vi "Fetch Measurement-Efficiency and Load Reg.vi"(8 "error in":errorcluster, 10 "Measure Call Context in":refnum<class "Measure Call Context.lvclass">, 11 "Efficency fetch measurement":T1={"Load,Source ON&OFF"=0, "Source Ganged Session Out"={"Ganged Config"=enum."Series", "Session List"=[], "Session Mode"=[], "Channel"=[]}, "Load Ganged Session Out"={"Ganged Config"=enum."Series", "Session List"=[], "Session Mode"=[], "Channel"=[]}, "Source sweep values"=[], "Source sweep points"=0, "Load sweep values"=[], "Load sweep points"=0, "Load ganged/single"=FALSE, "Source ganged/single"=FALSE, "Source channel name"="", "Load channel name"="", "Source session out"="", "Load session out"="", "measurement results"={"Source sweep points"=0, "Load sweep points"=0, "Voltage values"=[], "Efficiency"=[], "Ganged load currents"=[], "Ganged load voltages"=[], "Load voltage deviation"=[], "Status"="", "Eload status"=""}, "Nominal output voltage"=0.0, "Measurement timeout"=10.0}) -> (0 "error out":errorcluster, 3 "Efficency fetch measurement":T1={"Load,Source ON&OFF"=0, "Source Ganged Session Out"={"Ganged Config"=enum."Series", "Session List"=[], "Session Mode"=[], "Channel"=[]}, "Load Ganged Session Out"={"Ganged Config"=enum."Series", "Session List"=[], "Session Mode"=[], "Channel"=[]}, "Source sweep values"=[], "Source sweep points"=0, "Load sweep values"=[], "Load sweep points"=0, "Load ganged/single"=FALSE, "Source ganged/single"=FALSE, "Source channel name"="", "Load channel name"="", "Source session out"="", "Load session out"="", "measurement results"={"Source sweep points"=0, "Load sweep points"=0, "Voltage values"=[], "Efficiency"=[], "Ganged load currents"=[], "Ganged load voltages"=[], "Load voltage deviation"=[], "Status"="", "Eload status"=""}, "Nominal output voltage"=0.0, "Measurement timeout"=10.0})   [LabVIEW 2021, in "Eff And Load Reg_Channel Ganging.lvlib"]
doc: "This vi will fetch the measurement in different configuration for and calculate efficiency and load regulation."
uses:
  Eff And Load Reg_Channel Ganging.lvlib
  <vilib>/Plug-In SDKs/Measurements/Measure Call Context/Measure Call Context.lvclass
  Controls/Efficency fetch measurement control.ctl
  shared subVIs/ctl/NIDCPower_channel_ganging - ctl - ganged session.ctl
  shared subVIs/ctl/NIDCPower_channel_ganging - ctl - ganged config.ctl
  shared subVIs/ctl/NIDCPower_channel_ganging - ctl - channel mode.ctl
  Measurement Results.ctl
  <vilib>/Plug-In SDKs/Measurements/Measure Call Context/Accessor/Is Canceled.vi
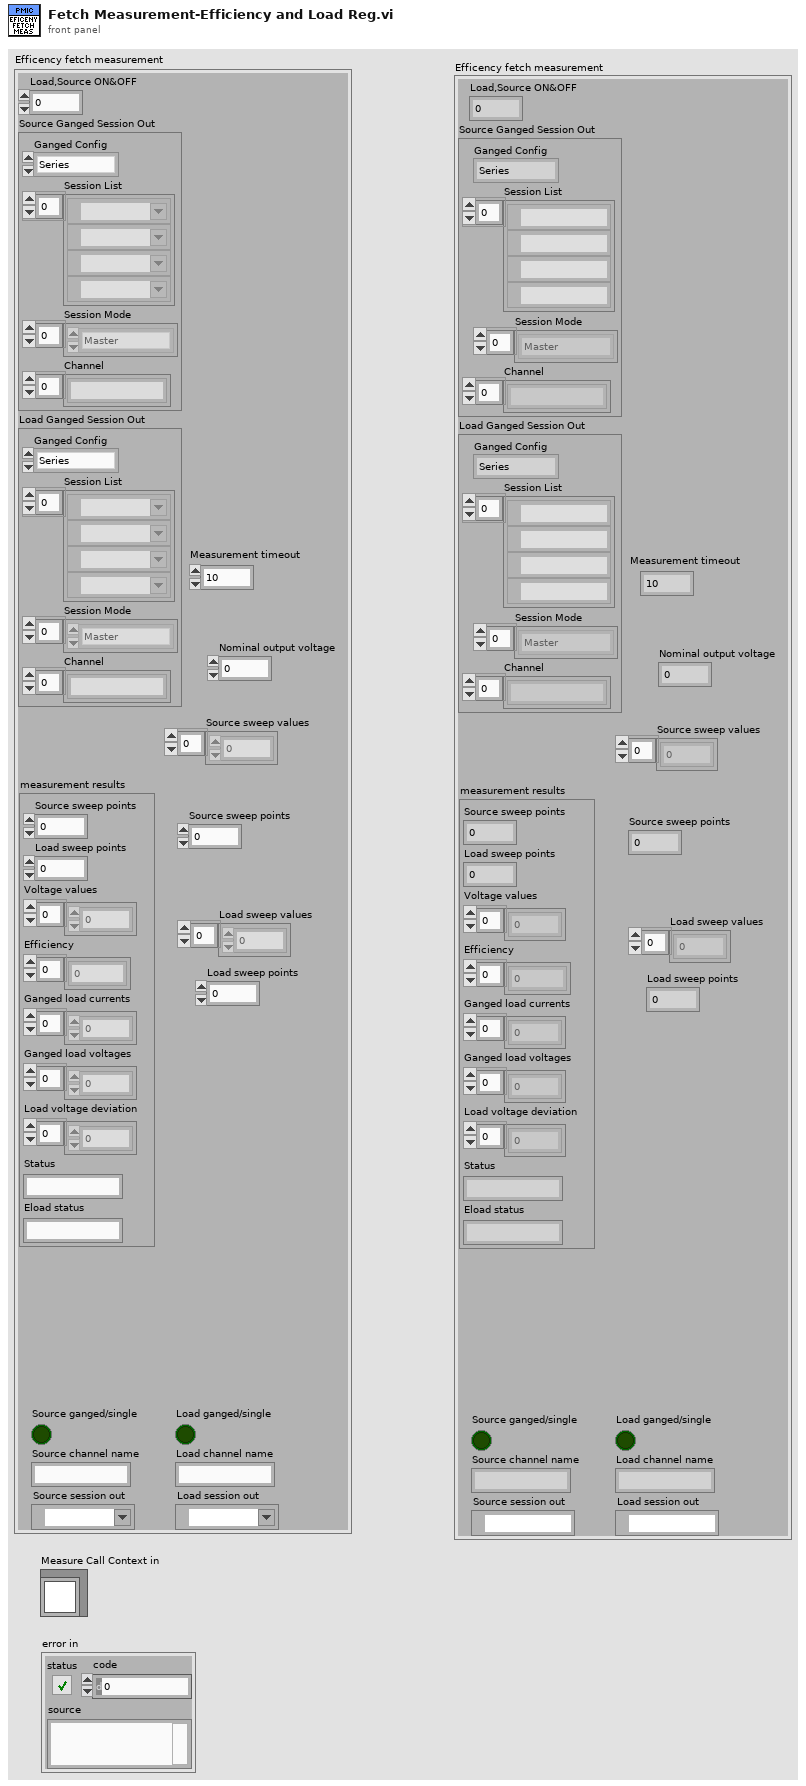
[diagram p1: front panel]
types:
  T1 = typedef "Eff And Load Reg_Channel Ganging.lvlib/Efficency fetch measurement control.ctl" = cluster{"Load,Source ON&OFF":u32, "Source Ganged Session Out":T2, "Load Ganged Session Out":T2, "Source sweep values":dbl[], "Source sweep points":i32, "Load sweep values":dbl[], "Load sweep points":i32, "Load ganged/single":bool, "Source ganged/single":bool, "Source channel name":string, "Load channel name":string, "Source session out":refnum<k15>, "Load session out":refnum<k15>, "measurement results":T5, "Nominal output voltage":dbl, "Measurement timeout":dbl}
  T2 = typedef "NIDCPower_channel_ganging - ctl - ganged session.ctl" = cluster{"Ganged Config":T3, "Session List":refnum<k15>[], "Session Mode":T4[], "Channel":string[]}
  T3 = typedef "NIDCPower_channel_ganging - ctl - ganged config.ctl" = enum32{"Series", "Parallel", "Manual"}
  T4 = typedef "NIDCPower_channel_ganging - ctl - channel mode.ctl" = enum32{"Master", "Slave", "Slave - Inverted"}
  T5 = typedef "Eff And Load Reg_Channel Ganging.lvlib/Measurement Results.ctl" = cluster{"Source sweep points":i32, "Load sweep points":i32, "Voltage values":dbl[], "Efficiency":dbl[], "Ganged load currents":dbl[], "Ganged load voltages":dbl[], "Load voltage deviation":dbl[], "Status":string, "Eload status":string}
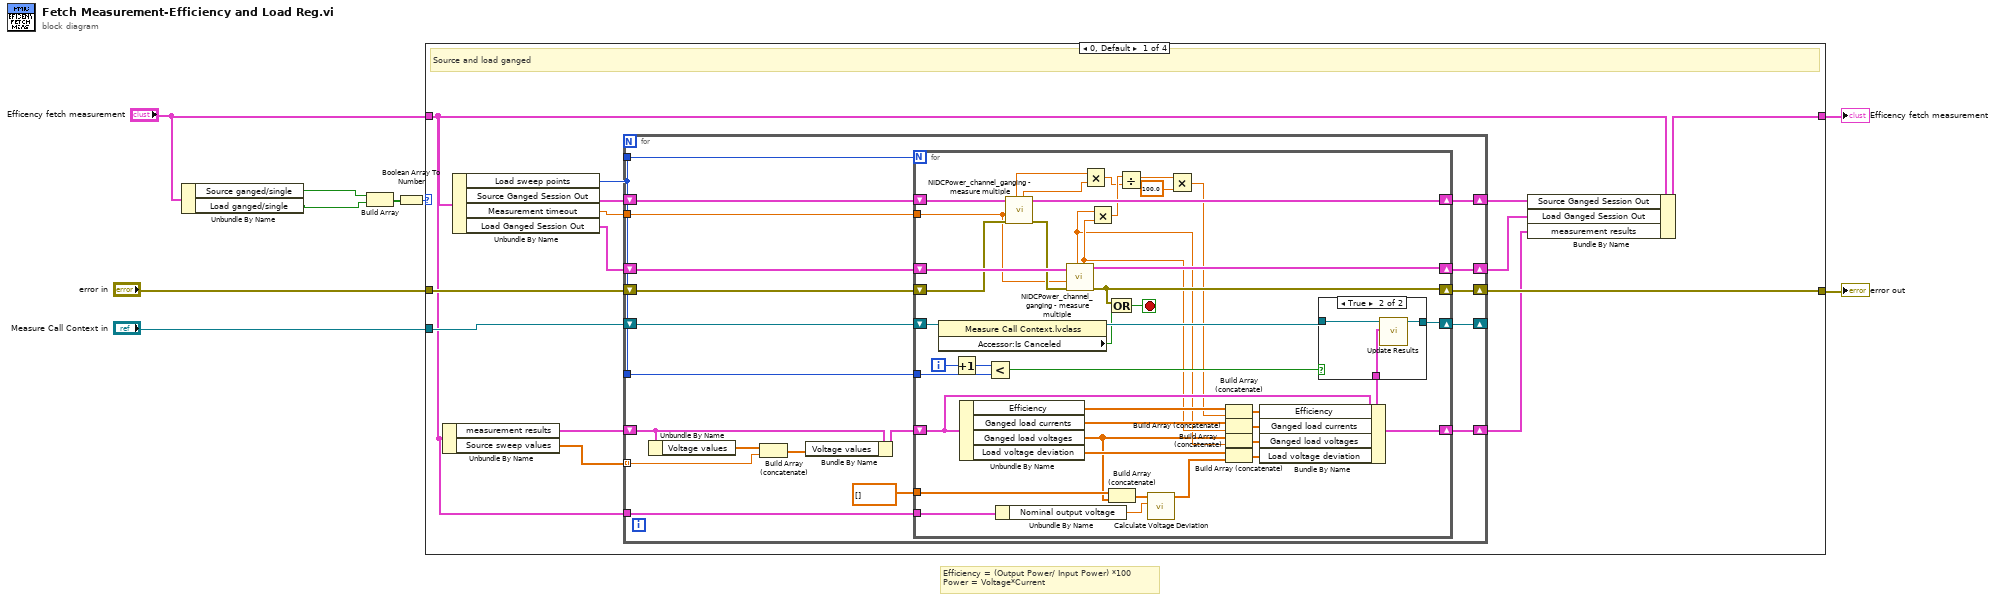
[diagram p0: block diagram]
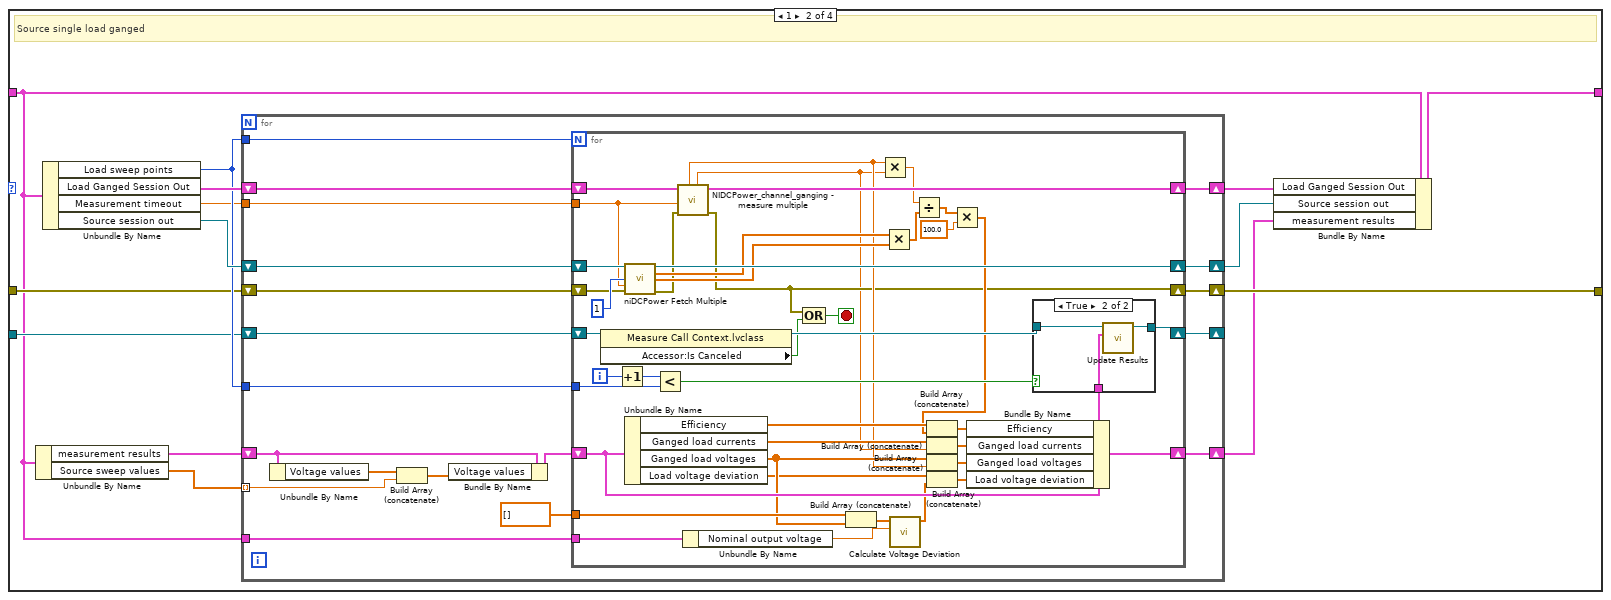
[diagram p3: hidden frame]
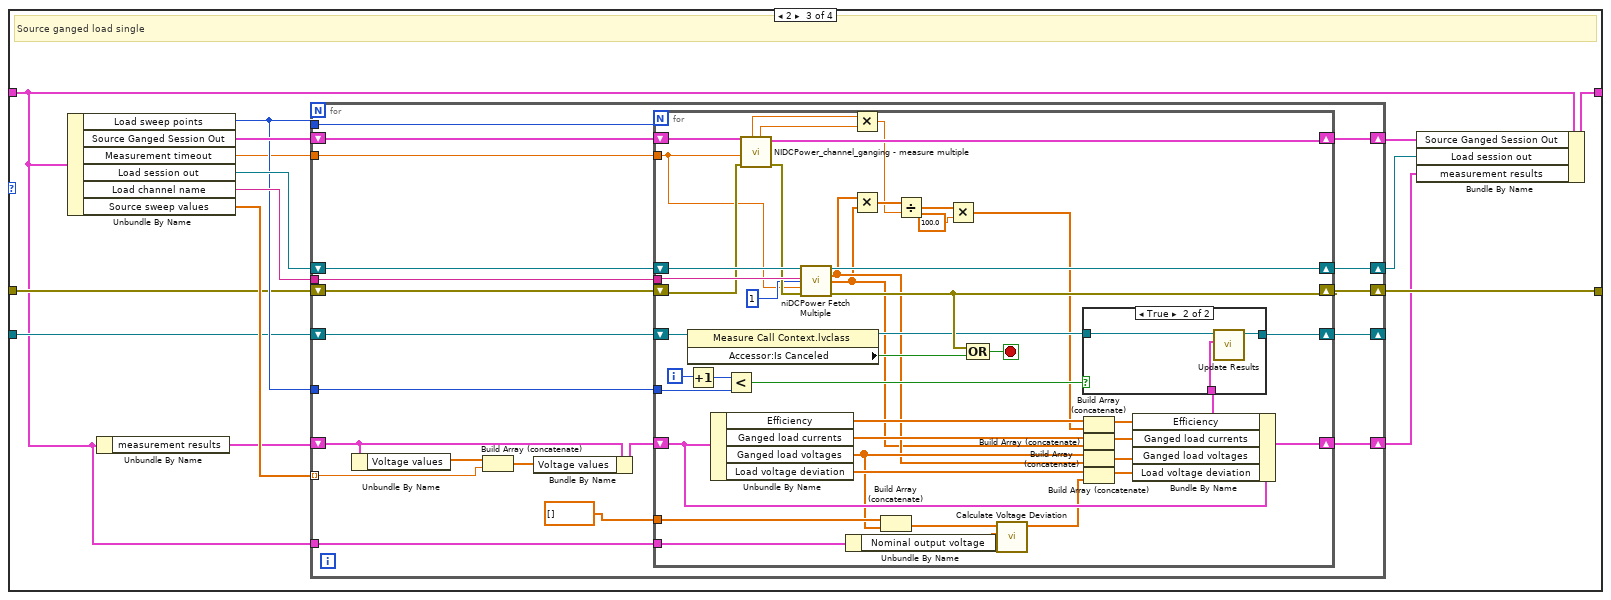
[diagram p5: hidden frame]
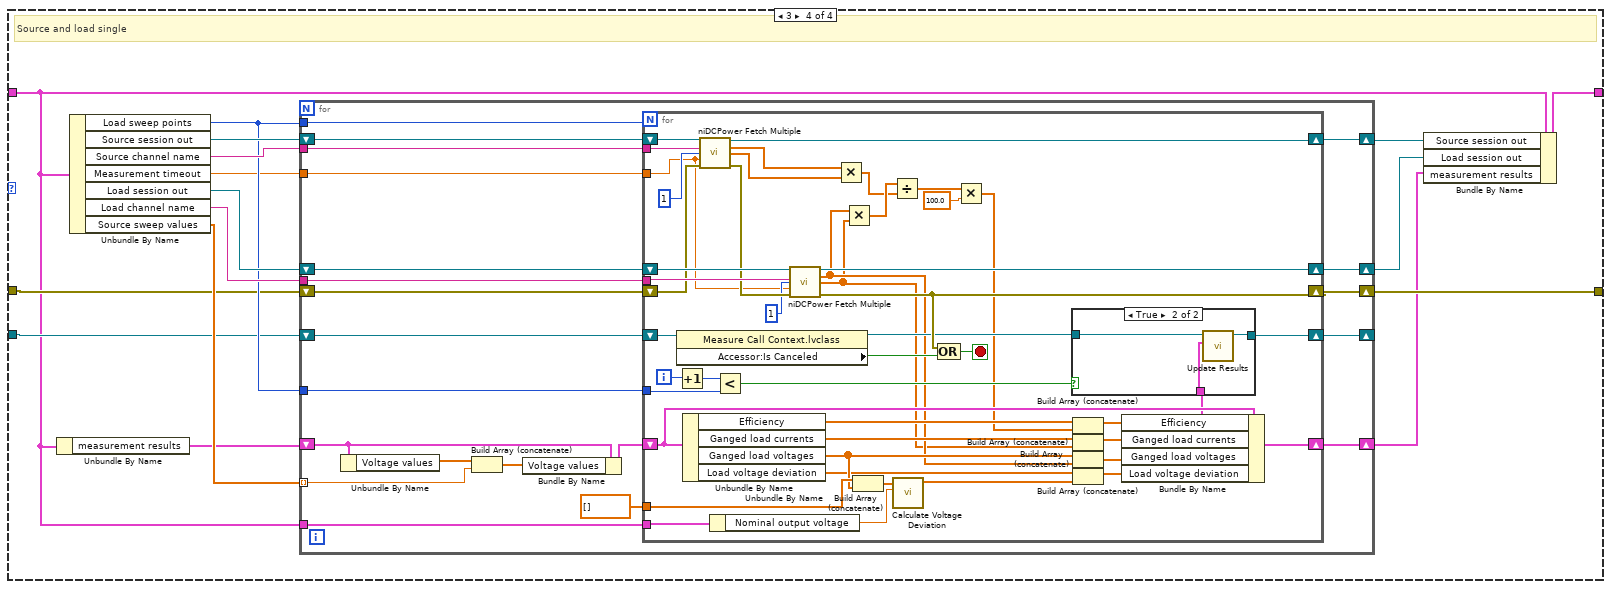
[diagram p7: hidden frame]
diagram:
  # "Efficiency = (Output Power/ Input Power) *100\nPower = Voltage*Current"
  n1 = Unbundle By Name("Efficency fetch measurement") -> ("Source ganged/single"=w6:bool, "Load ganged/single"=w5:bool)
  n2 = Build Array(w6, w5) -> (w3:bool[])
  n3 = Boolean Array To Number(Boolean array=w3) -> (number=w2:u32)
  n4 = case shown="0, Default" w2 {
    tunnel: "Efficency fetch measurement" -> [w12 w91 w169 w250]
    tunnel: [w22 w89 w172 w252] -> w1
    tunnel: "Measure Call Context in" -> [w15 w95 w175 w254]
    tunnel: [w14 w93 w173 w253] -> w8
    tunnel: "error in" -> [w13 w94 w176 w255]
    frame 0, Default {
      # "Source and load ganged"
      n5 = Unbundle By Name(w12) -> ("measurement results"=w16:T5, "Source sweep values"=w23:dbl[])
      n6 = Unbundle By Name(w12) -> ("Load sweep points"=w17:i32, "Source Ganged Session Out"=w18:T2, "Measurement timeout"=w10:dbl, "Load Ganged Session Out"=w19:T2)
      n7 = for {
        shift-right: [w41] -> w14
        shift-left: w13 -> [w42]
        shift-right: [w39] -> w21
        shift-left: w19 -> [w40]
        shift-right: [w37] -> w20
        shift-left: w18 -> [w38]
        shift-right: [w35] -> _
        shift-left: w15 -> [w36]
        shift-right: [w34] -> w11
        shift-left: w16 -> [w30]
        tunnel: w17 -> [w33]
        tunnel: w17 -> [w32]
        tunnel: w23 -> [w25] mode=indexing
        tunnel: w12 -> [w27]
        tunnel: w10 -> [w24]
        n8 = Unbundle By Name(w30) -> ("Voltage values"=w31:dbl[])
        n9 = Build Array (concatenate)(w31, w25) -> (w26:dbl[])
        n10 = Bundle By Name(cluster=w30, "Voltage values"=w26) -> (w29:T5)
        n11 = for {
          N: w32 -> [_]
          shift-right: [w72] -> w41
          shift-left: w42 -> [w81]
          shift-right: [w82] -> w39
          shift-left: w40 -> [w83]
          shift-right: [w78] -> w37
          shift-left: w38 -> [w79]
          shift-right: [w75] -> w35
          shift-left: w36 -> [w77]
          shift-right: [w70] -> w34
          shift-left: w29 -> [w71]
          tunnel: w33 -> [w66]
          tunnel: dbl[] [] ("Voltage measurements") -> [w51]
          tunnel: w27 -> [w48]
          tunnel: w24 -> [w45]
          i -> [w68]
          stop <- w74 stop-if-true
          n12 = property class="Measure Call Context.lvclass"(reference=w77) -> (reference out=w76:refnum<class "Measure Call Context.lvclass">, "Accessor:Is Canceled"=w73:bool)  [unwired: 1 in, 1 out]
          n13 = Increment(x=w68) -> (x+1=w69:i32)
          n14 = Unbundle By Name(w71) -> ("Efficiency"=w65:dbl[], "Ganged load currents"=w64:dbl[], "Ganged load voltages"=w47:dbl[], "Load voltage deviation"=w50:dbl[])
          n15 = Less?(x=w69, y=w66) -> (x < y?=w67:bool)
          n16 = Unbundle By Name(w48) -> ("Nominal output voltage"=w46:dbl)
          n17 = call "NIDCPower_channel_ganging - measure multiple.vi"("error in (no error)"=w81, "timeout (1.0)"=w45, "Ganged Session In"=w79) -> ("error out"=w80:errorcluster, "Ganged Session Out"=w78:T2, "ganged current measurement"=w56:dbl, "ganged voltage measurement"=w57:dbl)  [unwired: 1 in, 4 out]
          n18 = call "NIDCPower_channel_ganging - measure multiple.vi"("error in (no error)"=w80, "timeout (1.0)"=w45, "Ganged Session In"=w83) -> ("error out"=w72:errorcluster, "Ganged Session Out"=w82:T2, "ganged current measurement"=w55:dbl, "ganged voltage measurement"=w53:dbl)  [unwired: 1 in, 4 out]
          n19 = Multiply(x=w57, y=w56) -> (x*y=w43:dbl)
          n20 = Multiply(x=w53, y=w55) -> (x*y=w44:dbl)
          n21 = Build Array (concatenate)(w51, w47) -> (w52:dbl[])
          n22 = Compound Arithmetic op=OR(w72, w73) -> (w74:bool)
          n23 = Divide(x=w44, y=w43) -> (x/y=w63:dbl)
          n24 = call "Calculate Voltage Deviation.vi"("Nominal output voltage"=w46, "Voltage measurements"=w52) -> ("Load voltage deviation"=w49:dbl[])  [unwired: 9 in]
          n25 = Multiply(x=w63, y=100.0) -> (x*y=w54:dbl)
          n26 = Build Array (concatenate)(w65, w54) -> (w61:dbl[])
          n27 = Build Array (concatenate)(w64, w55) -> (w60:dbl[])
          n28 = Build Array (concatenate)(w47, w53) -> (w59:dbl[])
          n29 = Build Array (concatenate)(w50, w49) -> (w58:dbl[])
          n30 = Bundle By Name(cluster=w71, "Efficiency"=w61, "Ganged load currents"=w60, "Ganged load voltages"=w59, "Load voltage deviation"=w58) -> (w70:T5)
          n31 = case shown="True" w67 {
            tunnel: w70 -> [_ w87]
            tunnel: w76 -> [w84 w86]
            tunnel: [w84 w85] -> w75
            frame False {
            }
            frame True {
              n32 = call <vilib>:"Update Results.vi"("measurement results"=w87, "measure call context in"=w86) -> ("measure call context out"=w85:refnum<class "Measure Call Context.lvclass">)  [unwired: 8 in, 1 out]
            }
          }
        }
      }
      n33 = Bundle By Name(cluster=w12, "Source Ganged Session Out"=w20, "Load Ganged Session Out"=w21, "measurement results"=w11) -> (w22:T1)
    }
    frame 1 {
      # "Source single load ganged"
      n34 = Unbundle By Name(w91) -> ("measurement results"=w96:T5, "Source sweep values"=w101:dbl[])
      n35 = Unbundle By Name(w91) -> ("Load sweep points"=w97:i32, "Load Ganged Session Out"=w98:T2, "Measurement timeout"=w88:dbl, "Source session out"=w99:refnum<k15>)
      n36 = for {
        shift-right: [w119] -> w93
        shift-left: w94 -> [w120]
        shift-right: [w117] -> w92
        shift-left: w99 -> [w118]
        shift-right: [w115] -> w100
        shift-left: w98 -> [w116]
        shift-right: [w113] -> _
        shift-left: w95 -> [w114]
        shift-right: [w112] -> w90
        shift-left: w96 -> [w107]
        tunnel: w97 -> [w111]
        tunnel: w97 -> [w110]
        tunnel: w101 -> [w105] mode=indexing
        tunnel: w91 -> [w104]
        tunnel: w88 -> [w102]
        n37 = Unbundle By Name(w107) -> ("Voltage values"=w109:dbl[])
        n38 = Build Array (concatenate)(w109, w105) -> (w108:dbl[])
        n39 = Bundle By Name(cluster=w107, "Voltage values"=w108) -> (w106:T5)
        n40 = for {
          N: w110 -> [_]
          shift-right: [w124] -> w119
          shift-left: w120 -> [w126]
          shift-right: [w142] -> w117
          shift-left: w118 -> [w143]
          shift-right: [w161] -> w115
          shift-left: w116 -> [w162]
          shift-right: [w158] -> w113
          shift-left: w114 -> [w160]
          shift-right: [w152] -> w112
          shift-left: w106 -> [w155]
          tunnel: w111 -> [w146]
          tunnel: w104 -> [w130]
          tunnel: dbl[] [] ("Voltage measurements") -> [w129]
          tunnel: w102 -> [w121]
          i -> [w150]
          stop <- w157 stop-if-true
          n41 = property class="Measure Call Context.lvclass"(reference=w160) -> (reference out=w159:refnum<class "Measure Call Context.lvclass">, "Accessor:Is Canceled"=w156:bool)  [unwired: 1 in, 1 out]
          n42 = Increment(x=w150) -> (x+1=w151:i32)
          n43 = call <instrlib>:"niDCPower Fetch Multiple.vi"("instrument handle"=w143, "count (1)"=1, "timeout (1.0)"=w121, "error in (no error)"=w126) -> ("instrument handle out"=w142:refnum<k15>, "voltage measurements"=w136:dbl[], "current measurements"=w135:dbl[], "error out"=w125:errorcluster)  [unwired: 1 in, 7 out]
          n44 = Unbundle By Name(w155) -> ("Efficiency"=w145:dbl[], "Ganged load currents"=w144:dbl[], "Ganged load voltages"=w128:dbl[], "Load voltage deviation"=w122:dbl[])
          n45 = Less?(x=w151, y=w146) -> (x < y?=w149:bool)
          n46 = call "NIDCPower_channel_ganging - measure multiple.vi"("error in (no error)"=w125, "timeout (1.0)"=w121, "Ganged Session In"=w162) -> ("error out"=w124:errorcluster, "Ganged Session Out"=w161:T2, "ganged current measurement"=w123:dbl, "ganged voltage measurement"=w127:dbl)  [unwired: 1 in, 4 out]
          n47 = Unbundle By Name(w130) -> ("Nominal output voltage"=w133:dbl)
          n48 = Compound Arithmetic op=OR(w124, w156) -> (w157:bool)
          n49 = Build Array (concatenate)(w129, w128) -> (w132:dbl[])
          n50 = Multiply(x=w127, y=w123) -> (x*y=w140:dbl)
          n51 = Multiply(x=w136, y=w135) -> (x*y=w139:dbl[])
          n52 = call "Calculate Voltage Deviation.vi"("Nominal output voltage"=w133, "Voltage measurements"=w132) -> ("Load voltage deviation"=w131:dbl[])  [unwired: 9 in]
          n53 = Divide(x=w140, y=w139) -> (x/y=w138:dbl[])
          n54 = Build Array (concatenate)(w144, w123) -> (w153:dbl[])
          n55 = Build Array (concatenate)(w128, w127) -> (w148:dbl[])
          n56 = Build Array (concatenate)(w122, w131) -> (w147:dbl[])
          n57 = Multiply(x=w138, y=100.0) -> (x*y=w134:dbl[])
          n58 = Build Array (concatenate)(w145, w134) -> (w154:dbl[])
          n59 = Bundle By Name(cluster=w155, "Efficiency"=w154, "Ganged load currents"=w153, "Ganged load voltages"=w148, "Load voltage deviation"=w147) -> (w152:T5)
          n60 = case shown="True" w149 {
            tunnel: w152 -> [_ w166]
            tunnel: w159 -> [w163 w165]
            tunnel: [w163 w164] -> w158
            frame False {
            }
            frame True {
              n61 = call <vilib>:"Update Results.vi"("measurement results"=w166, "measure call context in"=w165) -> ("measure call context out"=w164:refnum<class "Measure Call Context.lvclass">)  [unwired: 8 in, 1 out]
            }
          }
        }
      }
      n62 = Bundle By Name(cluster=w91, "Load Ganged Session Out"=w100, "Source session out"=w92, "measurement results"=w90) -> (w89:T1)
    }
    frame 2 {
      # "Source ganged load single"
      n63 = Unbundle By Name(w169) -> ("Load sweep points"=w177:i32, "Source Ganged Session Out"=w181:T2, "Measurement timeout"=w167:dbl, "Load session out"=w180:refnum<k15>, "Load channel name"=w179:string, "Source sweep values"=w178:dbl[])
      n64 = Unbundle By Name(w169) -> ("measurement results"=w174:T5)
      n65 = for {
        tunnel: w179 -> [w195]
        tunnel: w177 -> [w194]
        shift-right: [w200] -> w173
        shift-left: w176 -> [w201]
        shift-right: [w198] -> w170
        shift-left: w181 -> [w197]
        shift-right: [w199] -> w171
        shift-left: w180 -> [w196]
        shift-right: [w192] -> _
        shift-left: w175 -> [w193]
        shift-right: [w185] -> w168
        shift-left: w174 -> [w189]
        tunnel: w178 -> [w190] mode=indexing
        tunnel: w177 -> [w191]
        tunnel: w169 -> [w183]
        tunnel: w167 -> [w182]
        n66 = Unbundle By Name(w189) -> ("Voltage values"=w186:dbl[])
        n67 = Build Array (concatenate)(w186, w190) -> (w187:dbl[])
        n68 = Bundle By Name(cluster=w189, "Voltage values"=w187) -> (w188:T5)
        n69 = for {
          N: w194 -> [_]
          tunnel: w195 -> [w243]
          shift-right: [w244] -> w199
          shift-left: w196 -> [w242]
          shift-right: [w240] -> w200
          shift-left: w201 -> [w222]
          shift-right: [w219] -> w198
          shift-left: w197 -> [w220]
          shift-right: [w231] -> w192
          shift-left: w193 -> [w237]
          shift-right: [w223] -> w185
          shift-left: w188 -> [w224]
          tunnel: w191 -> [w230]
          tunnel: dbl[] [] ("Voltage measurements") -> [w215]
          tunnel: w183 -> [w213]
          tunnel: w182 -> [w202]
          i -> [w238]
          stop <- w233 stop-if-true
          n70 = property class="Measure Call Context.lvclass"(reference=w237) -> (reference out=w232:refnum<class "Measure Call Context.lvclass">, "Accessor:Is Canceled"=w241:bool)  [unwired: 1 in, 1 out]
          n71 = Increment(x=w238) -> (x+1=w239:i32)
          n72 = Unbundle By Name(w224) -> ("Efficiency"=w234:dbl[], "Ganged load currents"=w229:dbl[], "Ganged load voltages"=w214:dbl[], "Load voltage deviation"=w235:dbl[])
          n73 = Less?(x=w239, y=w230) -> (x < y?=w228:bool)
          n74 = call "NIDCPower_channel_ganging - measure multiple.vi"("error in (no error)"=w222, "timeout (1.0)"=w202, "Ganged Session In"=w220) -> ("error out"=w221:errorcluster, "Ganged Session Out"=w219:T2, "ganged current measurement"=w207:dbl, "ganged voltage measurement"=w206:dbl)  [unwired: 1 in, 4 out]
          n75 = call <instrlib>:"niDCPower Fetch Multiple.vi"("instrument handle"=w242, "channel name"=w243, "count (1)"=1, "timeout (1.0)"=w202, "error in (no error)"=w221) -> ("instrument handle out"=w244:refnum<k15>, "voltage measurements"=w209:dbl[], "current measurements"=w208:dbl[], "error out"=w240:errorcluster)  [unwired: 7 out]
          n76 = Unbundle By Name(w213) -> ("Nominal output voltage"=w217:dbl)
          n77 = Multiply(x=w206, y=w207) -> (x*y=w203:dbl)
          n78 = Multiply(x=w209, y=w208) -> (x*y=w204:dbl[])
          n79 = Build Array (concatenate)(w215, w214) -> (w216:dbl[])
          n80 = Divide(x=w204, y=w203) -> (x/y=w211:dbl[])
          n81 = Multiply(x=w211, y=100.0) -> (x*y=w205:dbl[])
          n82 = Compound Arithmetic op=OR(w240, w241) -> (w233:bool)
          n83 = call "Calculate Voltage Deviation.vi"("Nominal output voltage"=w217, "Voltage measurements"=w216) -> ("Load voltage deviation"=w212:dbl[])  [unwired: 9 in]
          n84 = Build Array (concatenate)(w234, w205) -> (w227:dbl[])
          n85 = Build Array (concatenate)(w229, w208) -> (w226:dbl[])
          n86 = Build Array (concatenate)(w214, w209) -> (w236:dbl[])
          n87 = Build Array (concatenate)(w235, w212) -> (w225:dbl[])
          n88 = Bundle By Name(cluster=w224, "Efficiency"=w227, "Ganged load currents"=w226, "Ganged load voltages"=w236, "Load voltage deviation"=w225) -> (w223:T5)
          n89 = case shown="True" w228 {
            tunnel: w232 -> [w245 w248]
            tunnel: [w245 w247] -> w231
            tunnel: w223 -> [_ w246]
            frame False {
            }
            frame True {
              n90 = call <vilib>:"Update Results.vi"("measurement results"=w246, "measure call context in"=w248) -> ("measure call context out"=w247:refnum<class "Measure Call Context.lvclass">)  [unwired: 8 in, 1 out]
            }
          }
        }
      }
      n91 = Bundle By Name(cluster=w169, "Source Ganged Session Out"=w170, "Load session out"=w171, "measurement results"=w168) -> (w172:T1)
    }
    frame 3 {
      # "Source and load single"
      n92 = Unbundle By Name(w250) -> ("measurement results"=w258:T5)
      n93 = Unbundle By Name(w250) -> ("Load sweep points"=w259:i32, "Source session out"=w264:refnum<k15>, "Source channel name"=w263:string, "Measurement timeout"=w249:dbl, "Load session out"=w262:refnum<k15>, "Load channel name"=w261:string, "Source sweep values"=w260:dbl[])
      n94 = for {
        tunnel: w263 -> [w280]
        tunnel: w261 -> [w278]
        tunnel: w259 -> [w277]
        shift-right: [w284] -> w253
        shift-left: w255 -> [w285]
        shift-right: [w282] -> w256
        shift-left: w264 -> [w281]
        shift-right: [w283] -> w257
        shift-left: w262 -> [w279]
        shift-right: [w275] -> _
        shift-left: w254 -> [w276]
        shift-right: [w268] -> w251
        shift-left: w258 -> [w272]
        tunnel: w260 -> [w273] mode=indexing
        tunnel: w259 -> [w274]
        tunnel: w250 -> [w266]
        tunnel: w249 -> [w265]
        n95 = Unbundle By Name(w272) -> ("Voltage values"=w269:dbl[])
        n96 = Build Array (concatenate)(w269, w273) -> (w270:dbl[])
        n97 = Bundle By Name(cluster=w272, "Voltage values"=w270) -> (w271:T5)
        n98 = for {
          N: w277 -> [_]
          tunnel: w278 -> [w329]
          tunnel: w280 -> [w306]
          shift-right: [w330] -> w283
          shift-left: w279 -> [w328]
          shift-right: [w326] -> w284
          shift-left: w285 -> [w309]
          shift-right: [w305] -> w282
          shift-left: w281 -> [w307]
          shift-right: [w318] -> w275
          shift-left: w276 -> [w323]
          shift-right: [w310] -> w268
          shift-left: w271 -> [w311]
          tunnel: w274 -> [w317]
          tunnel: dbl[] [] ("Voltage measurements") -> [w301]
          tunnel: w266 -> [w297]
          tunnel: w265 -> [w286]
          i -> [w324]
          stop <- w320 stop-if-true
          n99 = property class="Measure Call Context.lvclass"(reference=w323) -> (reference out=w319:refnum<class "Measure Call Context.lvclass">, "Accessor:Is Canceled"=w327:bool)  [unwired: 1 in, 1 out]
          n100 = Increment(x=w324) -> (x+1=w325:i32)
          n101 = Unbundle By Name(w311) -> ("Efficiency"=w321:dbl[], "Ganged load currents"=w316:dbl[], "Ganged load voltages"=w300:dbl[], "Load voltage deviation"=w298:dbl[])
          n102 = call <instrlib>:"niDCPower Fetch Multiple.vi"("instrument handle"=w307, "channel name"=w306, "count (1)"=1, "timeout (1.0)"=w286, "error in (no error)"=w309) -> ("instrument handle out"=w305:refnum<k15>, "voltage measurements"=w291:dbl[], "current measurements"=w295:dbl[], "error out"=w308:errorcluster)  [unwired: 7 out]
          n103 = Unbundle By Name(w297) -> ("Nominal output voltage"=w296:dbl)
          n104 = Less?(x=w325, y=w317) -> (x < y?=w315:bool)
          n105 = call <instrlib>:"niDCPower Fetch Multiple.vi"("instrument handle"=w328, "channel name"=w329, "count (1)"=1, "timeout (1.0)"=w286, "error in (no error)"=w308) -> ("instrument handle out"=w330:refnum<k15>, "voltage measurements"=w294:dbl[], "current measurements"=w293:dbl[], "error out"=w326:errorcluster)  [unwired: 7 out]
          n106 = Multiply(x=w291, y=w295) -> (x*y=w287:dbl[])
          n107 = Multiply(x=w294, y=w293) -> (x*y=w288:dbl[])
          n108 = Build Array (concatenate)(w301, w300) -> (w299:dbl[])
          n109 = Divide(x=w288, y=w287) -> (x/y=w292:dbl[])
          n110 = call "Calculate Voltage Deviation.vi"("Nominal output voltage"=w296, "Voltage measurements"=w299) -> ("Load voltage deviation"=w302:dbl[])  [unwired: 9 in]
          n111 = Compound Arithmetic op=OR(w326, w327) -> (w320:bool)
          n112 = Multiply(x=w292, y=100.0) -> (x*y=w289:dbl[])
          n113 = Build Array (concatenate)(w321, w289) -> (w314:dbl[])
          n114 = Build Array (concatenate)(w316, w293) -> (w313:dbl[])
          n115 = Build Array (concatenate)(w300, w294) -> (w322:dbl[])
          n116 = Build Array (concatenate)(w298, w302) -> (w312:dbl[])
          n117 = Bundle By Name(cluster=w311, "Efficiency"=w314, "Ganged load currents"=w313, "Ganged load voltages"=w322, "Load voltage deviation"=w312) -> (w310:T5)
          n118 = case shown="True" w315 {
            tunnel: w319 -> [w331 w334]
            tunnel: [w331 w333] -> w318
            tunnel: w310 -> [_ w332]
            frame False {
            }
            frame True {
              n119 = call <vilib>:"Update Results.vi"("measurement results"=w332, "measure call context in"=w334) -> ("measure call context out"=w333:refnum<class "Measure Call Context.lvclass">)  [unwired: 8 in, 1 out]
            }
          }
        }
      }
      n120 = Bundle By Name(cluster=w250, "Source session out"=w256, "Load session out"=w257, "measurement results"=w251) -> (w252:T1)
    }
  }
  "error out" <- w8
  "Efficency fetch measurement" <- w1
